vi "pumpe.vi"() -> ()   [LabVIEW 2013]
panel:
  out "Driver Error":bool
  in  "Enable":bool
  in  "Fill/Empty SB":bool
  out "Motor Current[A]":dbl
  in  "PWM Duty Cycle (0-1)":dbl(slide) scale=0.0..1.0
  in  "stop":bool
  # "Richtungschalter"
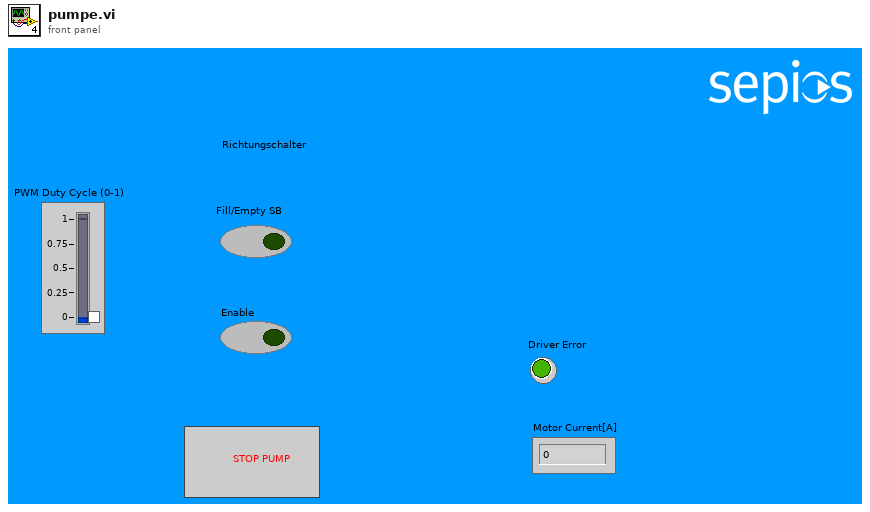
[diagram p1: front panel]
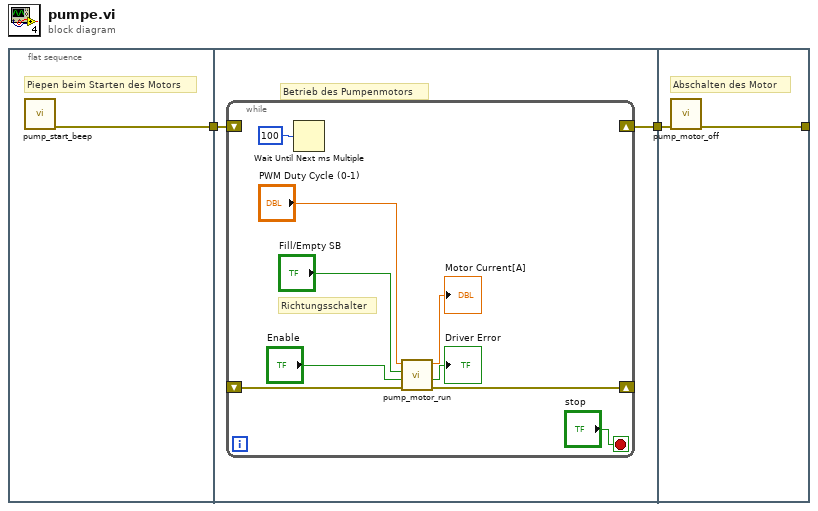
[diagram p0: block diagram]
diagram:
  n1 = flat-sequence {
    tunnel: [w3] -> w1
    tunnel: [w5] -> w2
    tunnel: w1 -> [w4]
    tunnel: w2 -> [w16]
    tunnel: [w15] -> _
    frame #0 {
      # "Piepen beim Starten des Motors"
      n2 = call "pump_start_beep.vi"() -> ("error out"=w3:errorcluster)  [unwired: 11 in]
    }
    frame #1 {
      # "Betrieb des Pumpenmotors"
      n3 = while {
        shift-right: [_] -> w5
        shift-left: w4 -> [_]
        shift-right: [w11] -> _
        shift-left: _ -> [w12]
        stop <- "stop" stop-if-true
        # "Richtungsschalter"
        n4 = Wait Until Next ms Multiple(millisecond multiple=u32 100) -> ()  [unwired: 1 out]
        n5 = call "pump_motor_run.vi"("error in (no error)"=w12, "Enable"="Enable", "Empty/Fill Swim Bladder"="Fill/Empty SB", "PWM Duty Cycle (0-1)"="PWM Duty Cycle (0-1)") -> ("error out"=w11:errorcluster, "Driver Error/Pump Motor off"=→"Driver Error":bool, "Motor Current[A]"=→"Motor Current[A]":dbl)  [unwired: 5 in]
      }
    }
    frame #2 {
      # "Abschalten des Motor"
      n6 = call "pump_motor_off.vi"("error in (no error)"=w16) -> ("error out"=w15:errorcluster)  [unwired: 10 in]
    }
  }
